vi "Create and Destroy Writer.vi"(8 "Error In":errorcluster) -> (0 "Error Out":errorcluster)   [LabVIEW 2017, in "Tests.lvlib"]
uses:
  Tests.lvlib
  src/LabPack/Public/Writer/Writer.lvclass
  <vilib>/addons/_JKI Toolkits/Caraya/classes/Test/Test.lvclass
  <vilib>/addons/_JKI Toolkits/Caraya/classes/Assert/Assert.lvclass
  src/LabPack/LabPack.lvlib
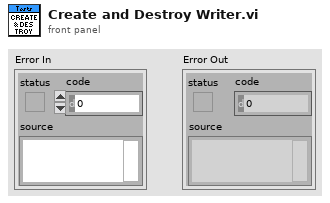
[diagram p1: front panel]
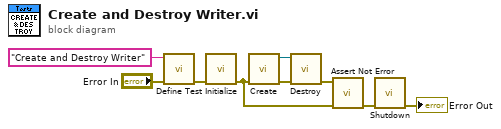
[diagram p0: block diagram]
diagram:
  n1 = call <vilib>:"Define Test.vi"("error in (no error)"="Error In", "Label (VI Title)"="Create and Destroy Writer") -> ("error out"=w5:errorcluster)  [unwired: 9 in]
  n2 = call "Initialize.vi"("Error In"=w5) -> ("Error Out"=w4:errorcluster)  [unwired: 10 in]
  n3 = call "Create.vi"("Error In"=w4) -> ("Error Out"=w8:errorcluster, "Writer"=w9:refnum<class "Writer.lvclass">)  [unwired: 9 in]
  n4 = call "Destroy.vi"("Error In"=w8, "Writer"=w9) -> ("Error Out"=w3:errorcluster)  [unwired: 9 in]
  n5 = call <vilib>:"Assert Not Error.vi"("error in (no error)"=w4, "Not Error?"=w3) -> ("error out"=w2:errorcluster)  [unwired: 9 in]
  n6 = call "Shutdown.vi"("Error In"=w2) -> ("Error Out"=→"Error Out":errorcluster)  [unwired: 10 in]
